vi "zadanie2.vi"() -> ()   [LabVIEW 2020]
panel:
  out "Temperatura obliczona na podstawie rezystancji":dbl
  in  "Wartoœæ rezystancji opornika platynowego":dbl
  # "Program oblicza wartoœæ temperatury na podstawie wartoœci rezystancji opornika platynowego"
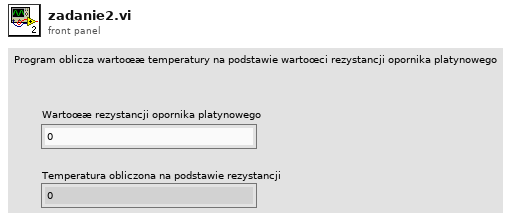
[diagram p1: front panel]
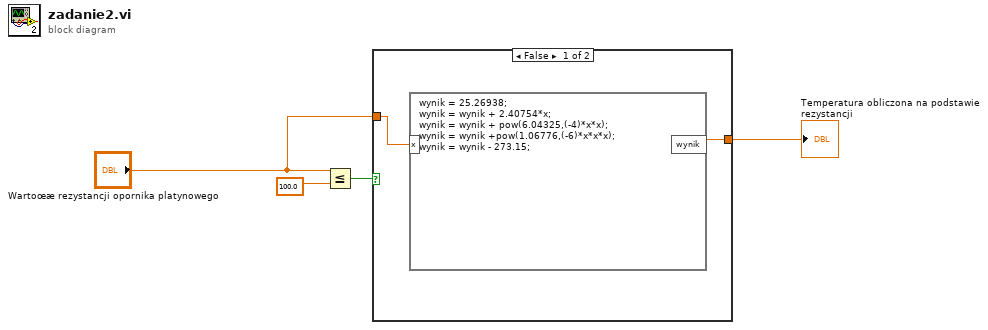
[diagram p0: block diagram]
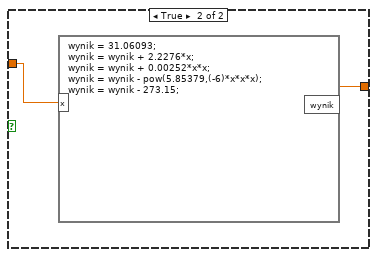
[diagram p2: hidden frame]
diagram:
  n1 = Less Or Equal?(x="Wartoœæ rezystancji opornika platynowego", y=100.0) -> (x <= y?=w4:bool)
  n2 = case shown="False" w4 {
    tunnel: "Wartoœæ rezystancji opornika platynowego" -> [w5 w7]
    tunnel: [w6 w8] -> w1
    frame False {
      n3 = formula code="wynik = 25.26938;\nwynik = wynik + 2.40754*x;\nwynik = wynik + pow(6.04325,(-4)*x*x);\nwynik = wynik +pow(1.06776,(-6)*x*x*x);\nwynik = wynik - 273.15;"("x"=w5) -> ("wynik"=w6:dbl)
    }
    frame True {
      n4 = formula code="wynik = 31.06093;\nwynik = wynik + 2.2276*x;\nwynik = wynik + 0.00252*x*x;\nwynik = wynik - pow(5.85379,(-6)*x*x*x);\nwynik = wynik - 273.15;"("x"=w7) -> ("wynik"=w8:dbl)
    }
  }
  "Temperatura obliczona na podstawie rezystancji" <- w1
